vi "DO Create.vi"(8 "error in (no error)":errorcluster, 10 "Digital Configuration Parameters":T1, 11 "TCP 380 in":refnum<class "TCP 380.lvclass">) -> (0 "error out":errorcluster, 3 "TCP 380 out":refnum<class "TCP 380.lvclass">)   [LabVIEW 2021, in "TCP 380.lvclass"]
uses:
  TCP 380.lvclass
  TCP 380.lvclass/TCP 380.ctl
  <vilib>/NathanCo/Digital-Tasks/Digital Output/Digital Output/Digital Output.lvclass
  <vilib>/NathanCo/Digital-Tasks/Utilities/Digital Configuration Parameters.ctl
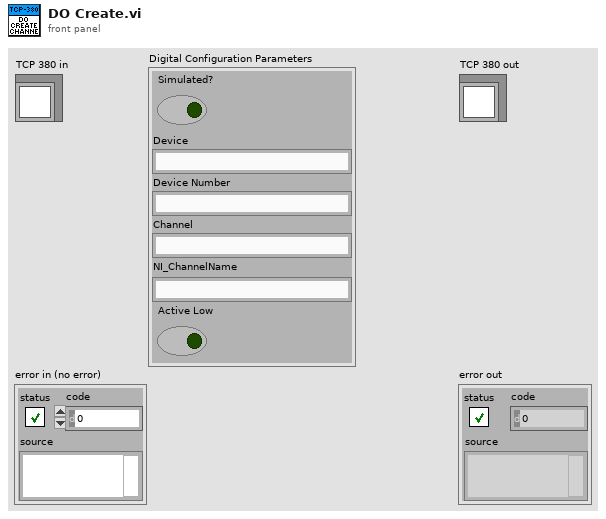
[diagram p1: front panel]
types:
  T1 = typedef "Digital Configuration Parameters.ctl" = cluster{"Simulated?":bool, "Device":string, "Device Number":string, "Channel":string, "NI_ChannelName":string, "Active Low":bool}
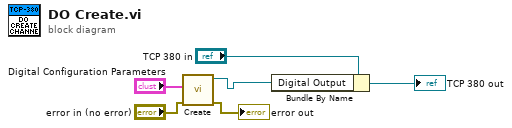
[diagram p0: block diagram]
diagram:
  n1 = call <vilib>:"Create.vi"("error in (no error)"="error in (no error)", "Digital Configuration Parameters"="Digital Configuration Parameters") -> ("error out"=→"error out":errorcluster, "Digital Output out"=w2:refnum<class "Digital Output.lvclass">)  [unwired: 8 in]
  n2 = Bundle By Name(cluster="TCP 380 in", "Digital Output"=w2) -> (→"TCP 380 out":refnum<class "TCP 380.lvclass">)
